vi "1A PWM Helper - Angle to Pulse Width.vi"(11 "ccw servo angle (radians)":dbl) -> (3 "pulse width (us)":u32)   [LabVIEW 2011]
doc: "Converts from counterclockwise angle in radians to pulse width in us. This VI is compatible with Hitec HS-4xx servo motors."
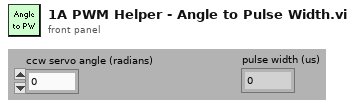
[diagram p1: front panel]
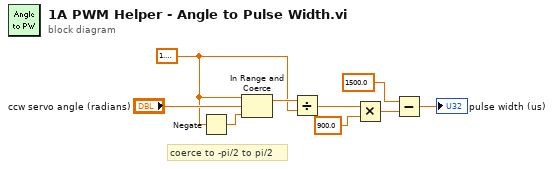
[diagram p0: block diagram]
diagram:
  w6 = 1.5707963267948966
  # "coerce to -pi/2 to pi/2"
  n1 = Negate(x=w6) -> (-x=w8:dbl)
  n2 = In Range and Coerce(upper limit=w6, x="ccw servo angle (radians)", lower limit=w8) -> (coerced(x)=w7:dbl)  [unwired: 1 out]
  n3 = Divide(x=w7, y=w6) -> (x/y=w5:dbl)
  n4 = Multiply(x=w5, y=900.0) -> (x*y=w3:dbl)
  n5 = Subtract(x=1500.0 ("y"), y=w3) -> (x-y=→"pulse width (us)":dbl)
